vi "MTMount_acceptCommand_configure.vi"(8 "error in (no error)":errorcluster, 11 "command_configure_Ctl":T1) -> (0 "error out":errorcluster, 2 "function return":i32, 3 "command_configure_Ctl out":T1)   [LabVIEW 2018, in "SALLV_MTMount.lvlib"]
doc: "int MTMount_shm_acceptCommand_configureLV(MTMount_command_configureLV *command_configure_Ctl );"
uses:
  SALLV_MTMount.lvlib
  DataTypes/command_configure.ctl
  SALLV_MTMount.so
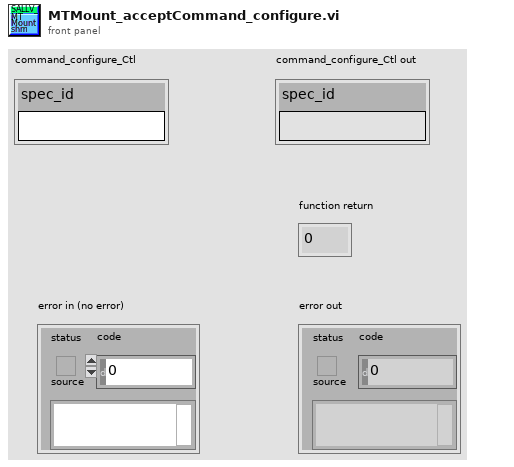
[diagram p1: front panel]
types:
  T1 = typedef "SALLV_MTMount.lvlib/command_configure.ctl" = cluster{"spec_id":string}
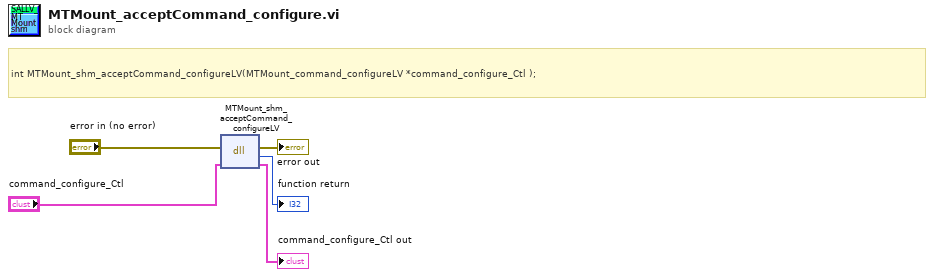
[diagram p0: block diagram]
diagram:
  # "int MTMount_shm_acceptCommand_configureLV(MTMount_command_configureLV *command_configure_Ctl );"
  n1 = dll-call lib="home/ttsai/Document/salApiMTMount/SALLV_MTMount/SALLV_MTMount.*" fn="MTMount_shm_acceptCommand_configureLV"(error in="error in (no error)", "command_configure_Ctl"="command_configure_Ctl") -> (error out=→"error out":errorcluster, →"function return":i32, "command_configure_Ctl"=→"command_configure_Ctl out":T1)  [unwired: 2 in, 1 out]
